vi "sv_Log View for Ratio (Array).vi"(7 "ratio units":enum16{"dB", "linear ratio", "%"}(ring), 8 "error in (no error)":errorcluster, 11 "linear ratio":dbl[](array[numeric]) format="%.3e") -> (0 "error out":errorcluster, 3 "converted ratio":dbl[](array[numeric]) format="%.3e", 5 "unit label":string)   [LabVIEW 2017, in "SoundVib_Distortion.lvlib"]
uses:
  <vilib>/addons/Sound and Vibration/svt_Distortion/SoundVib_Distortion.lvlib
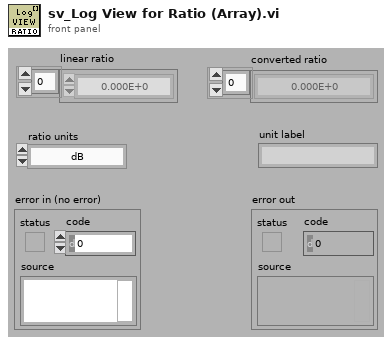
[diagram p1: front panel]
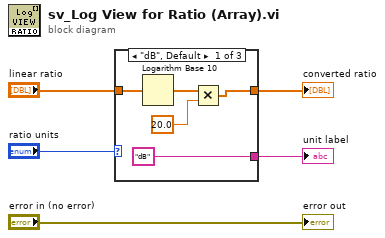
[diagram p0: block diagram]
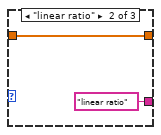
[diagram p2: hidden frame]
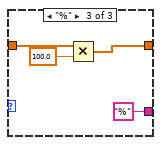
[diagram p3: hidden frame]
diagram:
  n1 = case shown="\"dB\", Default" "ratio units" {
    tunnel: [w7 w12 w14] -> w4
    tunnel: "linear ratio" -> [w10 w12 w16]
    tunnel: ["dB" "linear ratio" "%"] -> w3
    frame "dB", Default {
      n2 = Logarithm Base 10(1:w10) -> (0:w9:dbl[])
      n3 = Multiply(x=w9, y=20.0) -> (x*y=w7:dbl[])
    }
    frame "linear ratio" {
    }
    frame "%" {
      n4 = Multiply(x=w16, y=100.0) -> (x*y=w14:dbl[])
    }
  }
  "unit label" <- w3
  "converted ratio" <- w4
  "error out" <- "error in (no error)"
